vi "Is Tokenizer Error or Thrown.vi"(0 "Error":errorcluster) -> (1 "Thrown?":bool, 2 "Tokenizer Error?":bool)   [LabVIEW 2020, in "Stream.lvlib" / "URLPattern.lvclass"]
uses:
  URLPattern.lvclass
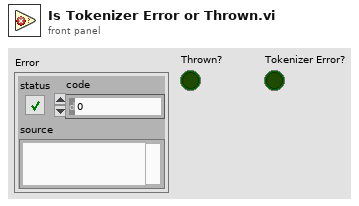
[diagram p1: front panel]
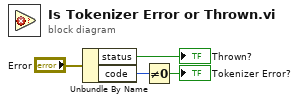
[diagram p0: block diagram]
diagram:
  n1 = Unbundle By Name("Error") -> ("status"=→"Thrown?":bool, "code"=w2:i32)
  n2 = Not Equal To 0?(x=w2) -> (x != 0?=→"Tokenizer Error?":bool)
